vi "GetType.vi"(8 "error in (no error)":errorcluster, 11 "Beep Msg":refnum<class "Beep Msg.lvclass">) -> (0 "error out":errorcluster, 2 "Data Sample":variant, 3 "Beep Msg":refnum<class "Beep Msg.lvclass">)   [LabVIEW 2016, in "CS++BeepActor.lvlib" / "Beep Msg.lvclass"]
uses:
  Beep Msg.lvclass
  Beep Msg.lvclass/Beep Msg.ctl
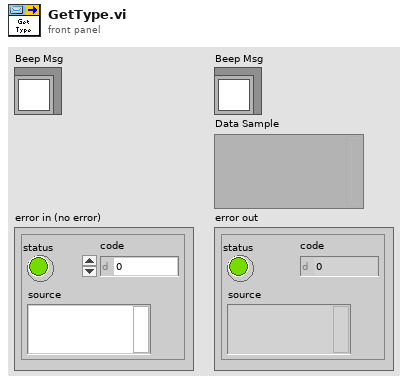
[diagram p1: front panel]
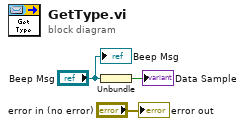
[diagram p0: block diagram]
diagram:
  n1 = Unbundle("Beep Msg") -> (→"Data Sample":bool)
  "error out" <- "error in (no error)"
  "Beep Msg" <- "Beep Msg"
